vi "oa_Update Current Time and Speed Segment.vi"(7 "reset? (F)":bool, 8 "error in (no error)":errorcluster, 10 "new spectrum available?":bool, 11 "segment status":T1) -> (0 "error out":errorcluster, 3 "segment status out":T1)   [LabVIEW 2017]
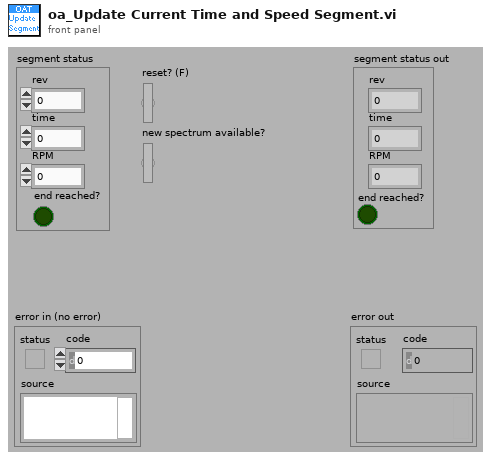
[diagram p1: front panel]
types:
  T1 = cluster{"rev":dbl, "time":dbl, "RPM":dbl, "end reached?":bool}
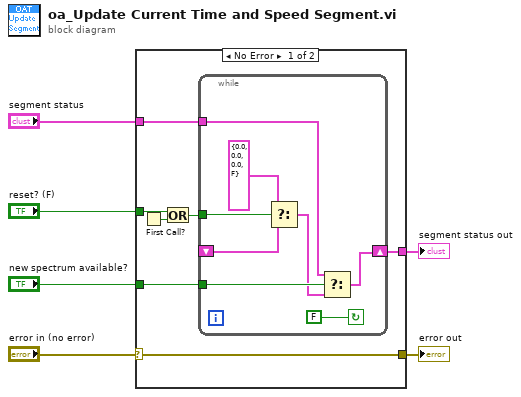
[diagram p0: block diagram]
diagram:
  n1 = case shown="No Error" "error in (no error)" {
    selector: "error in (no error)" -> [w13 w22]
    tunnel: [w13 w22] -> w5
    tunnel: "segment status" -> [w11 _]
    tunnel: "reset? (F)" -> [w9 _]
    tunnel: "new spectrum available?" -> [w12 _]
    tunnel: [w10 _] -> w1
    frame No Error {
      n2 = First Call?() -> (First Call?: T/F=w8:bool)
      n3 = Or(x=w9, y=w8) -> (x .or. y?=w7:bool)
      n4 = while {
        shift-right: [w16] -> w10
        shift-left: _ -> [w19]
        tunnel: w7 -> [w20]
        tunnel: w12 -> [w17]
        tunnel: w11 -> [w14]
        stop <- FALSE continue-if-true
        n5 = Select(t=T1 {"rev"=0.0, "time"=0.0, "RPM"=0.0, "end reached?"=FALSE} ("segment status"), s=w20, f=w19) -> (s? t:f=w15:T1)
        n6 = Select(t=w14, s=w17, f=w15) -> (s? t:f=w16:T1)
      }
    }
    frame Error {
    }
  }
  "error out" <- w5
  "segment status out" <- w1
